vi "Inverse Error Function.vi"(3 "x":dbl) -> (1 "inverf(x)":dbl)   [LabVIEW 2017, in "NI_AAL_MathFunc.lvlib"]
doc: "Computes the inverse of the error function associated with a normal distribution."
uses:
  <vilib>/gmath/NI_AAL_MathFunc.lvlib
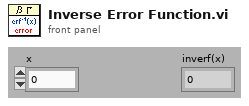
[diagram p1: front panel]
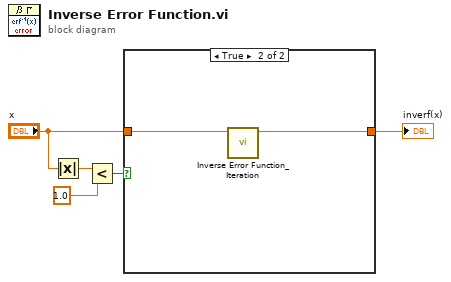
[diagram p0: block diagram]
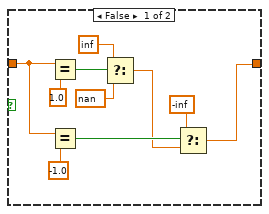
[diagram p2: hidden frame]
diagram:
  n1 = Absolute Value(x="x") -> (abs(x)=w5:dbl)
  n2 = Less?(x=w5, y=1.0) -> (x < y?=w3:bool)
  n3 = case shown="True" w3 {
    tunnel: "x" -> [w13 w17]
    tunnel: [w6 w16] -> w1
    frame False {
      n4 = Equal?(x=w13, y=1.0) -> (x = y?=w12:bool)
      n5 = Equal?(x=w13, y=-1.0) -> (x = y?=w9:bool)
      n6 = Select(t=inf, s=w12, f=nan) -> (s? t:f=w8:dbl)
      n7 = Select(t=-inf, s=w9, f=w8) -> (s? t:f=w6:dbl)
    }
    frame True {
      n8 = call <vilib>:"Inverse Error Function_Iteration.vi"("x"=w17) -> ("erfinv(x)"=w16:dbl)  [unwired: 10 in]
    }
  }
  "inverf(x)" <- w1
